vi "CSC_InitConfig1.vi"(8 "error in (no error)":errorcluster, 11 "C-Alex in":refnum<class "CableSerialChain.lvclass">) -> (0 "error out":errorcluster, 3 "C-Alex out":refnum<class "CableSerialChain.lvclass">)   [LabVIEW 2014, in "CableSerialChain.lvclass"]
uses:
  CableSerialChain.lvclass
  CableSerialChain.lvclass/CableSerialChain.ctl
  Body/PointOnBody.ctl
  Cable.ctl
  Body/Bodies.lvclass
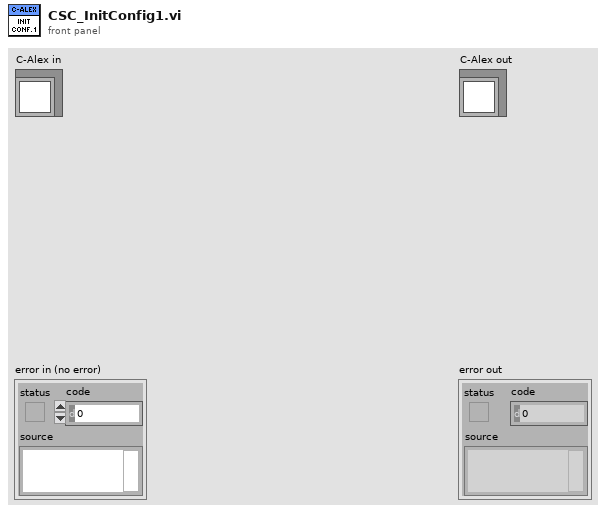
[diagram p1: front panel]
types:
  T1 = typedef "Bodies.lvclass/PointOnBody.ctl" = cluster{"Coord4":dbl[], "ID":i32}
  T2 = cluster{cluster{enum16{"Theta", "Alpha", "a", "d"}, dbl}[], "CoM_Pos":T1, "Mass(kg)":dbl}[]
  T3 = typedef "CableSerialChain.lvclass/Cable.ctl" = cluster{"RoutingPtsInLegCoSys":T1[], "Cable ID":i32}
  T4 = cluster{enum16{"Theta", "Alpha", "a", "d"}, dbl}[][]
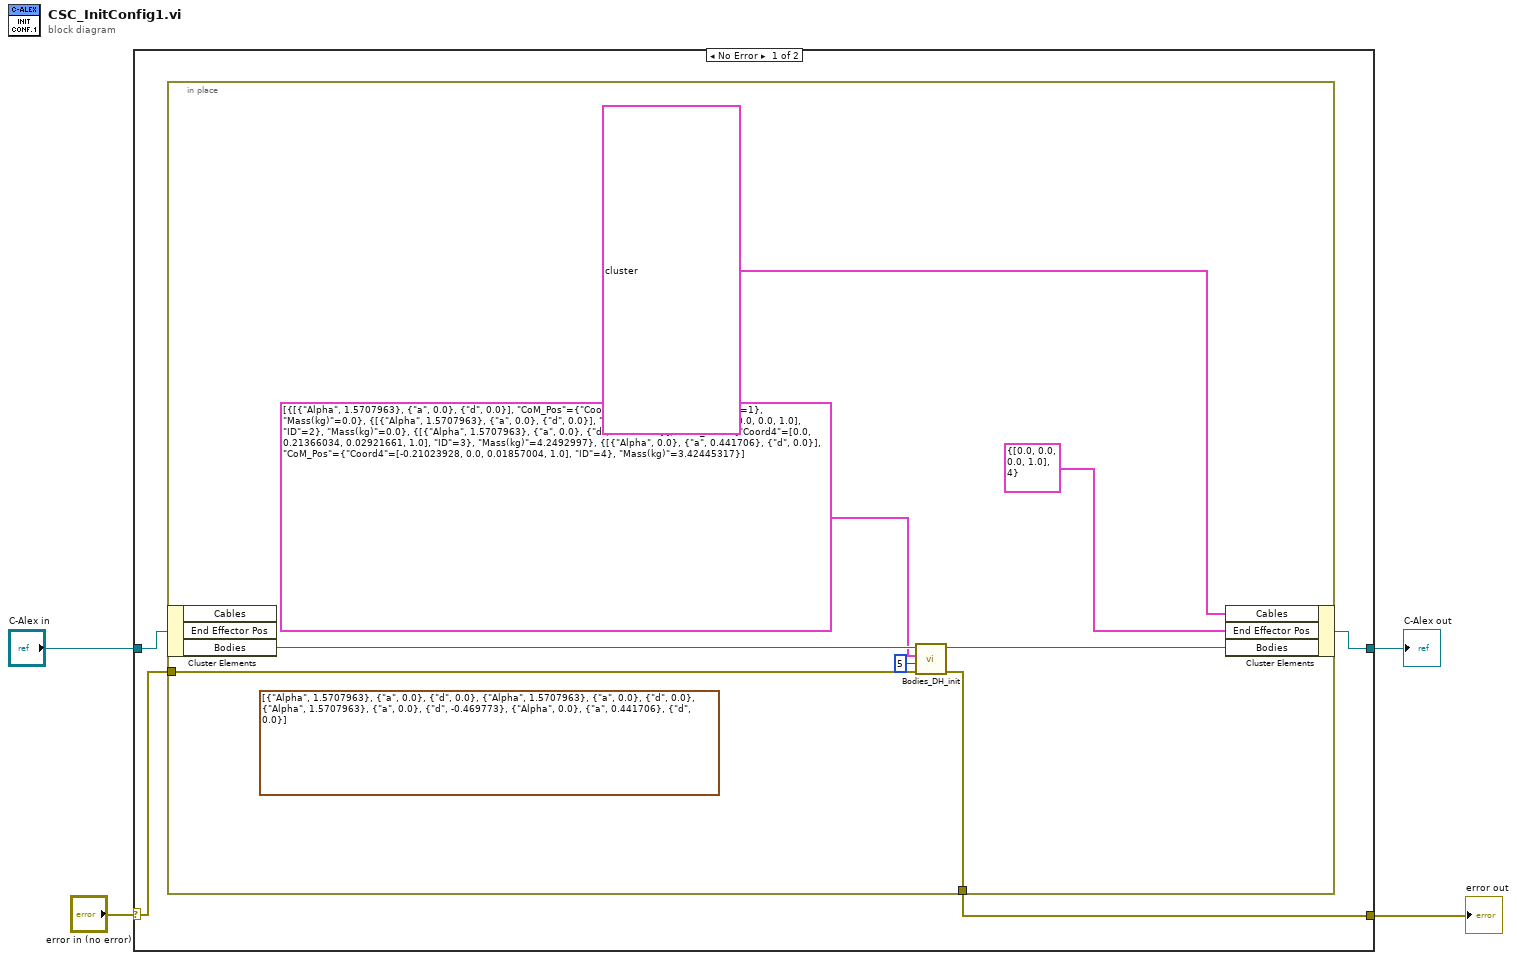
[diagram p0: block diagram]
diagram:
  n1 = case shown="No Error" "error in (no error)" {
    selector: "error in (no error)" -> [w7 w17]
    tunnel: [w5 w17] -> w3
    tunnel: [w6 w18] -> w1
    tunnel: "C-Alex in" -> [w8 w18]
    frame No Error {
      n2 = in-place {
        in-place-border: w7 -> [w15]
        in-place-border: [w11] -> w5
        (unwired) T4 [[{enum."Alpha", 1.5707963}, {enum."a", 0.0}, {enum."d", 0.0}], [{enum."Alpha", 1.5707963}, {enum."a", 0.0}, {enum."d", 0.0}], [{enum."Alpha", 1.5707963}, {enum."a", 0.0}, {enum."d", -0.469773}], [{enum."Alpha", 0.0}, {enum."a", 0.441706}, {enum."d", 0.0}]] ("KnownVar")
        n3 = in-place-cluster #1(w8) -> ("Bodies"=w16:refnum<class "Bodies.lvclass">)  [unwired: 2 out]
        n4 = call "Bodies_DH_init.vi"("error in (no error)"=w15, "Number of Bodies (Including Base)"=5, "KnownDHVars"=T2 [{[{enum."Alpha", 1.5707963}, {enum."a", 0.0}, {enum."d", 0.0}], "CoM_Pos"={"Coord4"=[0.0, 0.0, 0.0, 1.0], "ID"=1}, "Mass(kg)"=0.0}, {[{enum."Alpha", 1.5707963}, {enum."a", 0.0}, {enum."d", 0.0}], "CoM_Pos"={"Coord4"=[0.0, 0.0, 0.0, 1.0], "ID"=2}, "Mass(kg)"=0.0}, {[{enum."Alpha", 1.5707963}, {enum."a", 0.0}, {enum."d", -0.469773}], "CoM_Pos"={"Coord4"=[0.0, 0.21366034, 0.02921661, 1.0], "ID"=3}, "Mass(kg)"=4.2492997}, {[{enum."Alpha", 0.0}, {enum."a", 0.441706}, {enum."d", 0.0}], "CoM_Pos"={"Coord4"=[-0.21023928, 0.0, 0.01857004, 1.0], "ID"=4}, "Mass(kg)"=3.42445317}], "Body.lvclass In"=w16) -> ("error out"=w11:errorcluster, "Body.lvclass Out"=w14:refnum<class "Bodies.lvclass">)  [unwired: 6 in]
        n5 = in-place-cluster #1("Cables"=T3[] [{"RoutingPtsInLegCoSys"=[{"Coord4"=[-0.359321, 0.034925, 0.009174, 1.0], "ID"=0}, {"Coord4"=[-0.264188, 0.200787, 0.006608, 1.0], "ID"=3}, {"Coord4"=[-0.203581, -0.225948, 0.012563, 1.0], "ID"=4}], "Cable ID"=7}, {"RoutingPtsInLegCoSys"=[{"Coord4"=[-0.321287, 0.034925, 0.006933, 1.0], "ID"=0}, {"Coord4"=[-0.226279, 0.200787, 0.002798, 1.0], "ID"=3}], "Cable ID"=6}, {"RoutingPtsInLegCoSys"=[{"Coord4"=[0.359321, 0.034925, 0.009174, 1.0], "ID"=0}, {"Coord4"=[0.264188, 0.200787, 0.006608, 1.0], "ID"=3}, {"Coord4"=[-0.203581, 0.225948, 0.012563, 1.0], "ID"=4}], "Cable ID"=4}, {"RoutingPtsInLegCoSys"=[{"Coord4"=[0.321287, 0.034925, 0.006933, 1.0], "ID"=0}, {"Coord4"=[0.226279, 0.200787, 0.002798, 1.0], "ID"=3}], "Cable ID"=5}], "End Effector Pos"=T1 {"Coord4"=[0.0, 0.0, 0.0, 1.0], "ID"=4} ("Point"), "Bodies"=w14) -> (w6:refnum<class "CableSerialChain.lvclass">)
      }
    }
    frame Error {
    }
  }
  "error out" <- w3
  "C-Alex out" <- w1
